vi "Actor Core.vi"(8 "error in":errorcluster, 11 "Changing Panels in":refnum<class "Changing Panels.lvclass">) -> (0 "error out":errorcluster, 3 "Actor out":refnum<class "Actor.lvclass">)   [LabVIEW 2020, in "2. Basic Panel Actors.lvlib" / "Changing Panels.lvclass"]
doc: "The user interface for this panel.\n----\nCopyright: MGI 2016\nAuthor: Derek Trepanier"
uses:
  Changing Panels.lvclass
  C:/Program Files/National Instruments/LabVIEW 2020/vi.lib/MGI/Panel Manager/Panel Actor/Panel Actor/Panel Actor.lvclass
  <vilib>/ActorFramework/Actor/Actor.lvclass
  <vilib>/ActorFramework/Message Enqueuer/Message Enqueuer.lvclass
  Panel/Sample Panel.lvclass
  <vilib>/MGI/Panel Manager/Panel/Window Position/Reference Position/Size/Reference Size/Reference Size.lvclass/Reference Size.ctl
  <vilib>/ActorFramework/Message Enqueuer/Message Enqueuer.lvclass/Message Enqueuer.ctl
  <vilib>/MGI/Panel Manager/Panel/Window Position/Reference Position/Size/Reference Size/Reference Size.vi
  <vilib>/ActorFramework/Message Enqueuer/Enqueue.vi
  Description Panel/Description Panel.lvclass
  <vilib>/MGI/Panel Manager/Panel/Panel/Subpanel/Subpanel.lvclass
  C:/Program Files/National Instruments/LabVIEW 2020/vi.lib/MGI/Panel Manager/Panel/Panel/Panel.lvclass
  <vilib>/MGI/Panel Manager/Panel/Window Position/Reference Position/Size/Reference Size/Reference Size.lvclass
  C:/Program Files/National Instruments/LabVIEW 2020/vi.lib/MGI/Panel Manager/Panel/Window Position/Reference Position/Size/Size.lvclass
  <vilib>/MGI/Panel Manager/Panel/Window Position/Reference Position/Ref Display/Ref Display.lvclass
  C:/Program Files/National Instruments/LabVIEW 2020/vi.lib/MGI/Panel Manager/Panel/Window Position/Window Position.lvclass
  <vilib>/MGI/Panel Manager/Panel/Panel/Window/Window.lvclass
  <vilib>/ActorFramework/Stop Msg/Stop Msg.lvclass
  C:/Program Files/National Instruments/LabVIEW 2020/vi.lib/ActorFramework/Message/Message.lvclass
  <vilib>/MGI/Panel Manager/Panel/Panel/Subpanel/Subpanel.vi
  <vilib>/MGI/Panel Manager/Panel/Window Position/Reference Position/Ref Display/Ref Display.vi
  <vilib>/MGI/Panel Manager/Panel/Panel/Window/Window.vi
  <vilib>/ActorFramework/Message Priority Queue/Priority Enqueue.vi
  <vilib>/MGI/Panel Manager/Panel Actor/Panel Actor/Panel Actor.lvclass
  <vilib>/MGI/Panel Manager/Panel/Panel.lvlib
  <vilib>/MGI/Panel Manager/Panel Actor/Panel Actor Messages/Change Panel Msg/Change Panel Msg.lvclass
  <vilib>/MGI/Panel Manager/Panel Actor/Panel Actor Messages/Show Panel Msg/Show Panel Msg.lvclass
  C:/Program Files/National Instruments/LabVIEW 2020/vi.lib/MGI/Panel Manager/Panel/Window Position/Reference Position/Size/Reference Size/Reference Size.lvclass
  C:/Program Files/National Instruments/LabVIEW 2020/vi.lib/MGI/Panel Manager/Panel/Window Position/Reference Position/Reference Position.lvclass
  C:/Program Files/National Instruments/LabVIEW 2020/vi.lib/MGI/Panel Manager/Panel/Window Position/Reference Position/Ref Display/Ref Display.lvclass
panel:
  in  "Items":i32(listbox)
  in  "New Item":bool
  in  "Undock":bool
  # "Select an item to the left to view its panel"
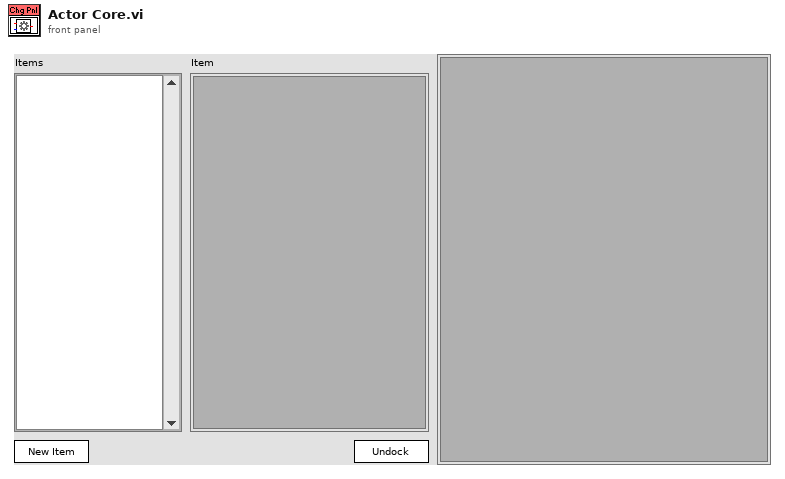
[diagram p1: front panel]
types:
  T1 = enum8{"Enabled", "Disabled", "Disabled and Grayed Out"}
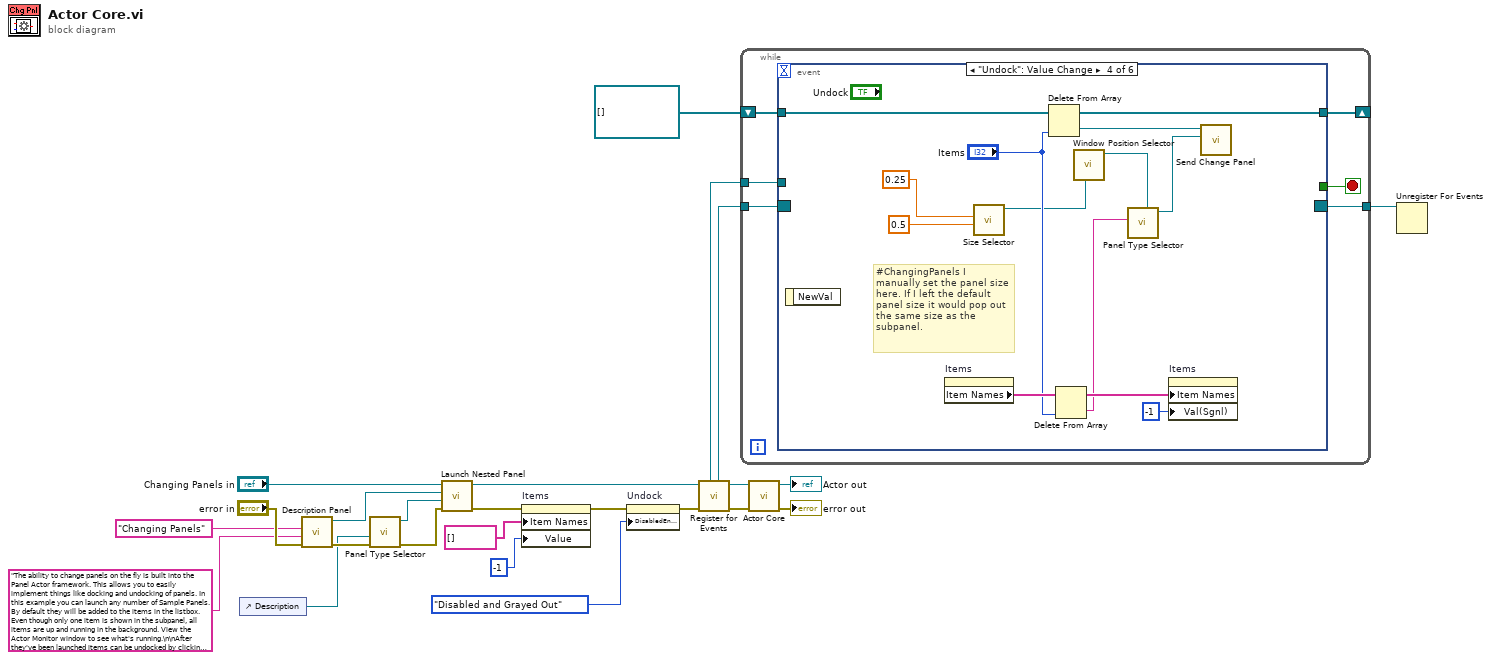
[diagram p0: block diagram]
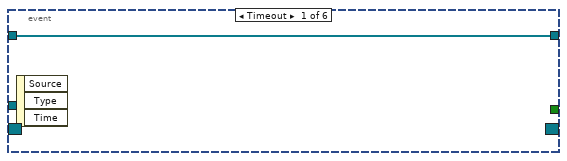
[diagram p2: hidden frame]
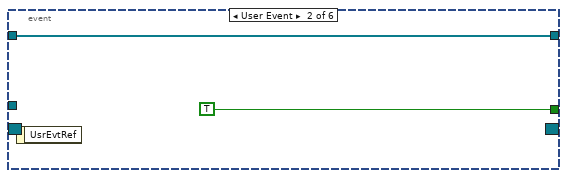
[diagram p3: hidden frame]
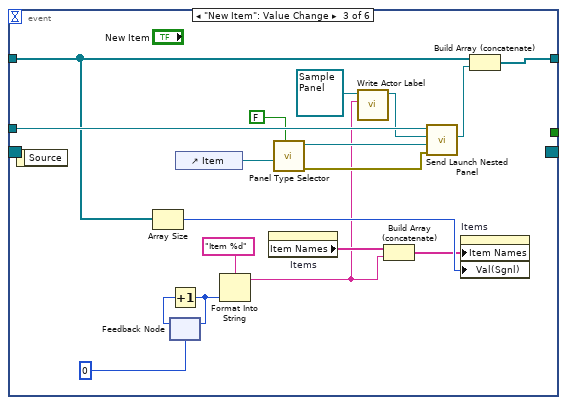
[diagram p4: hidden frame]
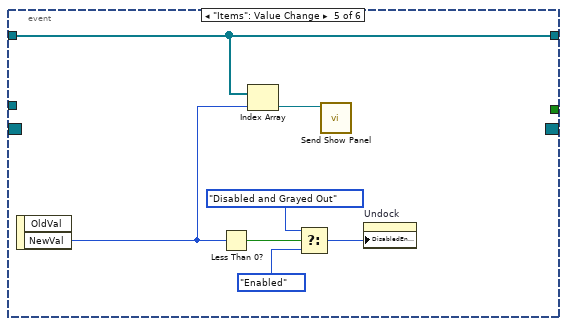
[diagram p5: hidden frame]
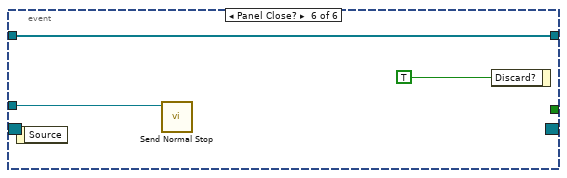
[diagram p6: hidden frame]
diagram:
  n1 = control-ref of="Description"() -> (w2:refnum<vi>)
  n2 = call "Description Panel.vi"("error in (no error)"="error in", "Description"="The ability to change panels on the fly is built into the Panel Actor framework. This allows you to easily implement things like docking and undocking of panels. In this example you can launch any number of Sample Panels. By default they will be added to the items in the listbox. Even though only one item is shown in the subpanel, all items are up and running in the background. View the Actor Monitor window to see what's running.\n\nAfter they've been launched items can be undocked by clicking the \"Undock\" button. This will send a \"Change Panel\" message to the panel actor with the new Window Panel object to use.\n\nThe Sample Panel Actor logs all panel events it encounters. Notice how the events that it receives when the panel changes. First it gets a Panel <b>Closed</b> Event. This is because the Subpanel Object is being closed. Next it gets a Panel <b>Initialized</b> Event. This is because the window was initialized. Finally it gets a Panel <b>Shown</b> Event.\n\nSee the #ChangingPanels bookmark for more info." ("Description Title"), "Description Title"="Changing Panels") -> ("error out"=w21:errorcluster, "Description Panel out"=w18:refnum<class "Description Panel.lvclass">)  [unwired: 7 in]
  n3 = call-poly <vilib>:"Panel Type Selector.vi"("Error In"=w21, "Sub Panel"=w2) -> ("Error Out"=w19:errorcluster, "Subpanel Out"=w20:refnum<class "Subpanel.lvclass">)  [unwired: 8 in]
  n4 = call <vilib>:"Launch Nested Panel.vi"("error in (no error)"=w19, "Panel"=w20, "Nested Panel Actor"=w18, "Panel Actor in"="Changing Panels in") -> ("error out"=w8:errorcluster, "Panel Actor out"=w13:refnum<class "Changing Panels.lvclass">)  [unwired: 4 in, 2 out]
  n5 = property on="Items" class="LstBox (strict)"(error in=w8, "Item Names"=string[] [], "Value"=-1 ("Items")) -> (error out=w5:errorcluster)  [unwired: 1 in, 1 out]
  n6 = property on="Undock" class="Bool"(error in=w5, "DisabledEnum"=T1."Disabled and Grayed Out" ("Disabled")) -> (error out=w4:errorcluster)  [unwired: 1 in, 1 out]
  n7 = call <vilib>:"Register for Events.vi"("Error In"=w4, "Panel Actor in"=w13) -> ("Error Out"=w14:errorcluster, "Panel Actor out"=w12:refnum<class "Changing Panels.lvclass">, "Pnl Actor"=w11:refnum<event-registration>, "Self Enqueuer"=w10:refnum<class "Message Enqueuer.lvclass">)  [unwired: 6 in]
  n8 = while {
    tunnel: w11 -> [w30]
    tunnel: w10 -> [w28]
    shift-right: [w26] -> _
    shift-left: refnum<class "Message Enqueuer.lvclass">[] [] -> [w27]
    tunnel: [w25] -> w1
    stop <- w29 stop-if-true
    n9 = event shown="[3] \"Undock\": Value Change" {
      selector: w30 -> [_ _ _ _ _ _]
      dyn-events: [_ _ _ _ _ _] -> w25
      timeout: _ -> [_ _ _ _ _ _]
      tunnel: [_ TRUE _ _ _ _] -> w29
      tunnel: w28 -> [_ _ w49 _ _ w73]
      tunnel: w27 -> [w31 w32 w44 w64 w67 w72]
      tunnel: [w31 w32 w50 w63 w67 w72] -> w26
      event Timeout {
        n10 = event-data() -> ()  [unwired: 1 in, 3 out]
      }
      event User Event {
        n11 = event-data() -> ()  [unwired: 1 in, 1 out]
      }
      event "New Item": Value Change {
        n12 = event-data() -> ()  [unwired: 1 in, 1 out]
        n13 = Array Size(array=w44) -> (size(s)=w39:i32)
        n14 = feedback #1(0) -> (w42:i32)
        n15 = Increment(x=w42) -> (x+1=w40:i32)
        n16 = feedback-in #1(w40) -> ()
        n17 = control-ref of="Item"() -> (w51:refnum<vi>)
        n18 = Format Into String(format string="Item %d", w40) -> (resulting string=w35:string)  [unwired: 2 in, 1 out]
        n19 = property on="Items" class="LstBox (strict)"() -> ("Item Names"=w37:string[])  [unwired: 2 in, 2 out]
        n20 = call-poly <vilib>:"Panel Type Selector.vi"("Autoshow? (T)"=FALSE, "Sub Panel"=w51) -> ("Error Out"=w45:errorcluster, "Subpanel Out"=w46:refnum<class "Subpanel.lvclass">)  [unwired: 8 in]
        n21 = call-dynamic "Write Actor Label.vi"("Actor Label"=w35, "Monitored Actor in"=refnum<class "Sample Panel.lvclass"> refnum ("2. Basic Panel Actors.lvlib:Sample Panel.lvclass")) -> ("Monitored Actor out"=w36:refnum<class "Sample Panel.lvclass">)  [unwired: 8 in, 1 out]
        n22 = Build Array (concatenate)(w37, w35) -> (w38:string[])
        n23 = call <vilib>:"Send Launch Nested Panel.vi"("Error In"=w45, "Panel"=w46, "Nested Panel Actor"=w36, "Self Enqueuer in"=w49) -> ("Nested Actor's Enqueuer"=w48:refnum<class "Message Enqueuer.lvclass">)  [unwired: 6 in, 1 out]
        n24 = property on="Items" class="LstBox (strict)"("Item Names"=w38, "Val(Sgnl)"=w39) -> ()  [unwired: 2 in, 2 out]
        n25 = Build Array (concatenate)(w44, w48) -> (w50:refnum<class "Message Enqueuer.lvclass">[])
      }
      event "Undock": Value Change {
        # "#ChangingPanels I manually set the panel size here. If I left the default panel size it would pop out the same size as the subpanel."
        n26 = event-data() -> ()  [unwired: 1 in, 1 out]
        n27 = property on="Items" class="LstBox (strict)"() -> ("Item Names"=w58:string[])  [unwired: 2 in, 2 out]
        n28 = call-poly <vilib>:"Size Selector.vi"("Height Scale"=0.5 ("Width Scale"), "Width Scale"=0.25) -> ("Static Out"=w54:refnum<class "Reference Size.lvclass">)  [unwired: 8 in, 1 out]
        n29 = Delete From Array(array=w64, index="Items") -> (deleted portion=w62:refnum<class "Message Enqueuer.lvclass">, array with subset deleted=w63:refnum<class "Message Enqueuer.lvclass">[])  [unwired: 1 in]
        n30 = Delete From Array(array=w58, index="Items") -> (deleted portion=w55:string, array with subset deleted=w57:string[])  [unwired: 1 in]
        n31 = call-poly <vilib>:"Window Position Selector.vi"("Size"=w54) -> ("Ref Display out"=w60:refnum<class "Ref Display.lvclass">)  [unwired: 9 in, 1 out]
        n32 = call-poly <vilib>:"Panel Type Selector.vi"("Window Position"=w60, "Default Title"=w55) -> ("Window out"=w61:refnum<class "Window.lvclass">)  [unwired: 8 in, 1 out]
        n33 = property on="Items" class="LstBox (strict)"("Item Names"=w57, "Val(Sgnl)"=-1 ("Value (Signaling)")) -> ()  [unwired: 2 in, 2 out]
        n34 = call <vilib>:"Send Change Panel.vi"("New Panel"=w61, "Message Enqueuer in"=w62) -> ()  [unwired: 8 in, 2 out]
      }
      event "Items": Value Change {
        n35 = event-data() -> ("NewVal"=w66:i32)  [unwired: 1 in, 1 out]
        n36 = Less Than 0?(x=w66) -> (x < 0?=w71:bool)
        n37 = Index Array(array=w67, index=w66) -> (element=w65:refnum<class "Message Enqueuer.lvclass">)
        n38 = Select(t=T1."Disabled and Grayed Out" ("Disabled"), s=w71, f=T1."Enabled" ("Disabled")) -> (s? t:f=w68:T1)
        n39 = call <vilib>:"Send Show Panel.vi"("Message Enqueuer in"=w65) -> ()  [unwired: 9 in, 2 out]
        n40 = property on="Undock" class="Bool"("DisabledEnum"=w68) -> ()  [unwired: 2 in, 2 out]
      }
      event Panel Close? {
        n41 = event-data() -> ()  [unwired: 1 in, 1 out]
        n42 = call <vilib>:"Send Normal Stop.vi"("Message Enqueuer"=w73) -> ()  [unwired: 10 in, 1 out]
        n43 = event-data("Discard?"=TRUE) -> ()  [unwired: 1 in, 1 out]
      }
    }
  }
  n44 = call-parent "Actor Core.vi"("error in"=w14, "Panel Actor in"=w12) -> ("error out"=→"error out":errorcluster, "Actor out"=→"Actor out":refnum<class "Actor.lvclass">)  [unwired: 8 in]
  n45 = Unregister For Events(event registration refnum=w1) -> ()  [unwired: 1 in, 1 out]
